vi "Test Multiple Doors API.vi"() -> ()   [LabVIEW 2018]
uses:
  Door/Door.lvclass
  Timed Door.lvclass
  C:/GitClones/LGP5-Resources/LVOOP/Interfaces/Timed Door/Classes/Door/Door.lvclass
  Set Target Time (seconds).vi
panel:
  out "error out":errorcluster
  in  "Create New Door":bool
  in  "Door Type":enum32{"Door", "Timed Door"}(radio)
  in  "Timed Door Target Time (seconds)":dbl=5.0
  in  "Door Switches":enum32{"Open Door", "Close Door"}[](array[radio])
  out "Door":u16[](array[ring])
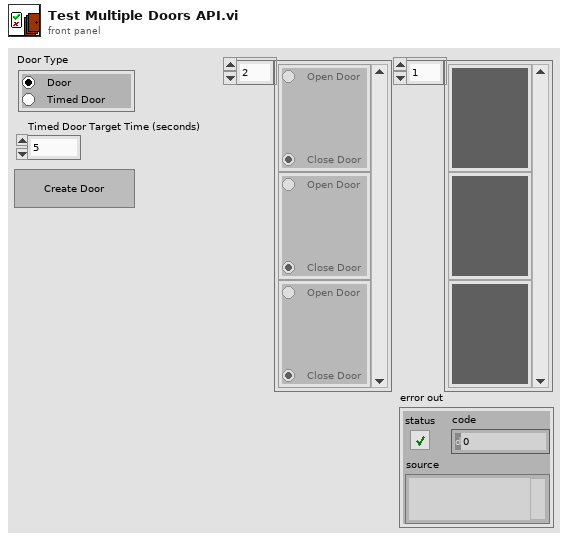
[diagram p1: front panel]
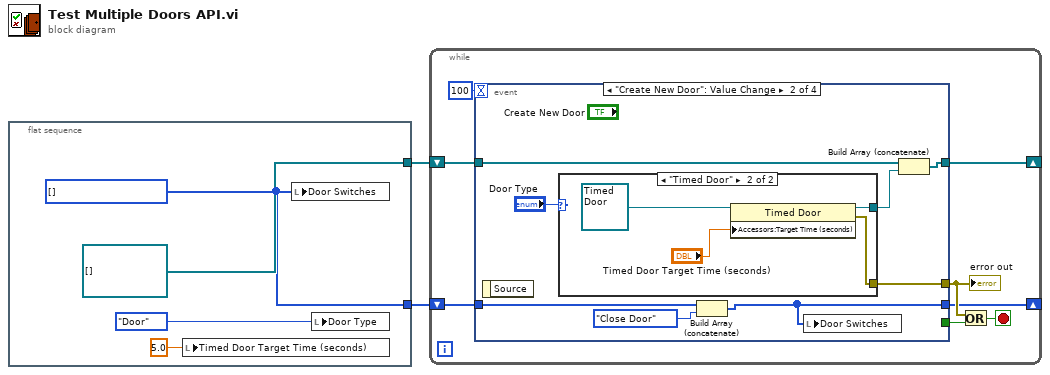
[diagram p0: block diagram]
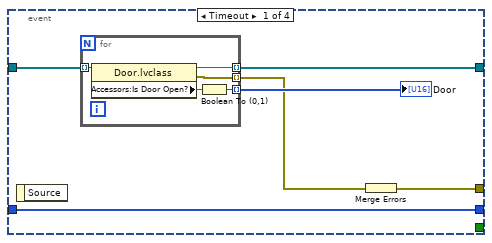
[diagram p2: hidden frame]
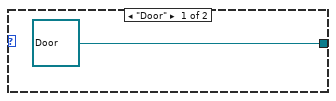
[diagram p3: hidden frame]
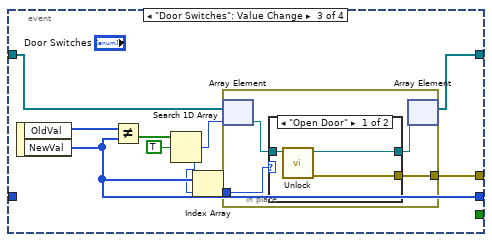
[diagram p4: hidden frame]
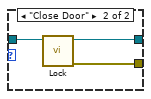
[diagram p5: hidden frame]
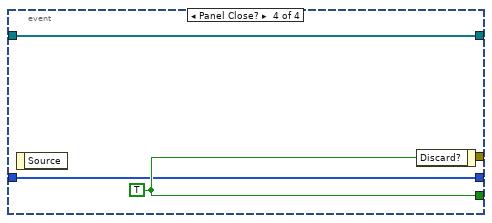
[diagram p6: hidden frame]
diagram:
  n1 = flat-sequence {
    tunnel: [refnum<class "Door.lvclass">[] [] ("Array")] -> w2
    tunnel: [w3] -> w1
    frame #0 {
      w3 = enum32{"Open Door", "Close Door"}[] [] items=["Open Door", "Close Door"] ("Door Switch")
      n2 = local write "Timed Door Target Time (seconds)"(5.0 ("Timed Door Target Time (seconds)")) -> ()
      n3 = local write "Door Switches"(w3) -> ()
      n4 = local write "Door Type"(enum32{"Door", "Timed Door"}."Door" ("Door Type")) -> ()
    }
  }
  n5 = while {
    shift-right: [w10] -> _
    shift-left: w2 -> [w12]
    shift-right: [w8] -> _
    shift-left: w1 -> [w9]
    stop <- w7 stop-if-true
    n6 = event shown="[1] \"Create New Door\": Value Change" {
      selector: _ -> [_ _ _ _]
      dyn-events: _ -> [_ _ _ _]
      timeout: 100 -> [_ _ _ _]
      tunnel: w12 -> [w18 w33 w43 w59]
      tunnel: [_ _ _ w60] -> w11
      tunnel: [w19 w32 w44 w59] -> w10
      tunnel: w9 -> [w17 w29 _ w58]
      tunnel: [w17 w27 w42 w58] -> w8
      tunnel: [w15 w26 w39 _] -> w14
      event Timeout {
        n7 = event-data() -> ()  [unwired: 1 in, 1 out]
        n8 = for {
          tunnel: [w24] -> w20 mode=indexing
          tunnel: [w23] -> w19 mode=indexing
          tunnel: w18 -> [w22] mode=indexing
          tunnel: [w21] -> w16 mode=indexing
          n9 = property class="Door.lvclass"(reference=w22) -> (reference out=w23:refnum<class "Door.lvclass">, error out=w21:errorcluster, "Accessors:Is Door Open?"=w25:bool)  [unwired: 1 in]
          n10 = Boolean To (0,1)(Boolean=w25) -> (0, 1=w24:i16)
        }
        "Door" <- w20
        n11 = Merge Errors(w16) -> (w15:errorcluster)
      }
      event "Create New Door": Value Change {
        n12 = event-data() -> ()  [unwired: 1 in, 1 out]
        n13 = case shown="\"Timed Door\"" "Door Type" {
          tunnel: [refnum<class "Door.lvclass"> refnum ("Door.lvclass") w37] -> w30
          tunnel: [_ w35] -> w26
          frame "Door" {
          }
          frame "Timed Door" {
            n14 = property class="Timed Door"(reference=refnum<class "Timed Door.lvclass"> refnum ("Timed Door.lvclass"), "Accessors:Target Time (seconds)"="Timed Door Target Time (seconds)") -> (reference out=w37:refnum<class "Timed Door.lvclass">, error out=w35:errorcluster)  [unwired: 1 in]
          }
        }
        n15 = Build Array (concatenate)(w29, enum32{"Open Door", "Close Door"}."Close Door" ("Door Switch")) -> (w27:enum32{"Open Door", "Close Door"}[])
        n16 = local write "Door Switches"(w27) -> ()
        n17 = Build Array (concatenate)(w33, w30) -> (w32:refnum<class "Door.lvclass">[])
      }
      event "Door Switches": Value Change {
        n18 = event-data() -> ("OldVal"=w47:enum32{"Open Door", "Close Door"}[], "NewVal"=w42:enum32{"Open Door", "Close Door"}[])  [unwired: 1 in]
        n19 = Not Equal?(x=w47, y=w42) -> (x != y?=w46:bool[])
        n20 = Search 1D Array(1D array=w46, element=TRUE) -> (index of element=w41:i32)  [unwired: 1 in]
        n21 = Index Array(array=w42, index=w41) -> (element=w40:enum32{"Open Door", "Close Door"})
        n22 = in-place {
          in-place-border: w40 -> [w49]
          in-place-border: [w48] -> w39
          n23 = in-place-array #1(w43, w41) -> (w51:refnum<class "Door.lvclass">)
          n24 = case shown="\"Open Door\"" w49 {
            tunnel: w51 -> [w54 w57]
            tunnel: [w53 w56] -> w50
            tunnel: [w52 w55] -> w48
            frame "Open Door" {
              n25 = call-dynamic "Unlock.vi"("Door in"=w54) -> ("error out"=w52:errorcluster, "Door out"=w53:refnum<class "Door.lvclass">)  [unwired: 9 in]
            }
            frame "Close Door" {
              n26 = call-dynamic "Lock.vi"("Door in"=w57) -> ("error out"=w55:errorcluster, "Door out"=w56:refnum<class "Door.lvclass">)  [unwired: 9 in]
            }
          }
          n27 = in-place-array #1(w50) -> (w44:refnum<class "Door.lvclass">[])  [unwired: 1 out]
        }
      }
      event Panel Close? {
        w60 = TRUE ("Discard?")
        n28 = event-data() -> ()  [unwired: 1 in, 1 out]
        n29 = event-data("Discard?"=w60) -> ()  [unwired: 1 in, 1 out]
      }
    }
    "error out" <- w14
    n30 = Or(x=w14, y=w11) -> (x .or. y?=w7:bool)
  }
